vi "Quick Test.vi"() -> ()   [LabVIEW 2010]
uses:
  <vilib>/SwitchExecutive/nise.llb/niSE Multiconnect Mode Enum.ctl
panel:
  in  "Load All Channels":bool
  in  "DMM to DVDD":bool
  in  "SMU1 to VRECT":bool
  in  "stop":bool
  in  "SMU3 to VBAT + BATT SIM":bool
  in  "SMU3 to VBAT":bool
  in  "JTAG DVDD POWER":bool
  in  "JTAG DATA":bool
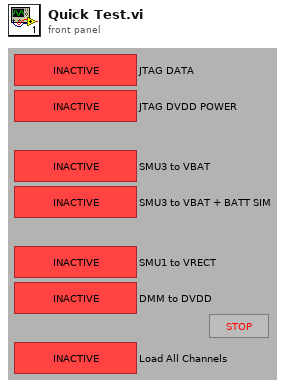
[diagram p1: front panel]
types:
  T1 = typedef "niSE Multiconnect Mode Enum.ctl" = i32
  T2 = typedef "niSE SessionRefnum.ctl" = refnum<k1>
  T3 = enum16{"--Disconnect All--", "Connect PulseGen to CH1", "Connect PulseGen to CH2", "Connect PulseGen to CH3", "Connect PulseGen to CH4", "Connect PulseGen to CH5", "Connect PulseGen to CH6", "Connect PulseGen to CH7", "Connect PulseGen to CH8", "Connect PulseGen to CH9", "Connect PulseGen to CH10", "Connect PulseGen to CH11", "Connect PulseGen to CH12", "Connect PulseGen to CH13", "Connect PulseGen to CH14", "Connect PulseGen to CH15", "Connect PulseGen to CH16", "Connect PulseGen to CH17", "Connect PulseGen to CH18", "Connect PulseGen to CH19", "Connect PulseGen to CH20", "Connect PulseGen to CH21", "Connect PulseGen to CH22", "Connect PulseGen to CH23", "Connect PulseGen to CH24", "Connect PulseGen to CH25", "Set MAG_SW", "Set Dynamic Load", "Set Expansion Trigger", "Trigger Positive Pulse", "Trigger Negative Pulse", "Set MSP Magic Pin", "Set BAT_EN", "Connect MSP_ACLK to CTR", "Connect MSP_MCLK to CTR", "Connect MSP_DIG_TST_OUT to CTR", "Connect STIM_SCK to CTR", "Connect STIM_CLK to CTR", "Connect SMU2 to Magnet", "Magnet Enable", "Cap Short", "Connect Positive Pulse to Pulse Bus", "Connect Negative Pulse to Pulse Bus", "Connect JTAG", "Connect JTAG DVDD Power", "RF Attach", "Connect SMU3 to VBAT", "Connect SMU3 Soft Start", "Connect ARB to Charge Coil", "Connect ARB to Matrix", "Connect CTR to Matrix", "DMM_I Short", "DMM_I 1000 Ohm", "DMM_I 100 Ohm", "DMM_I 10 Ohm", "Connect CH25 to DUT GND"}
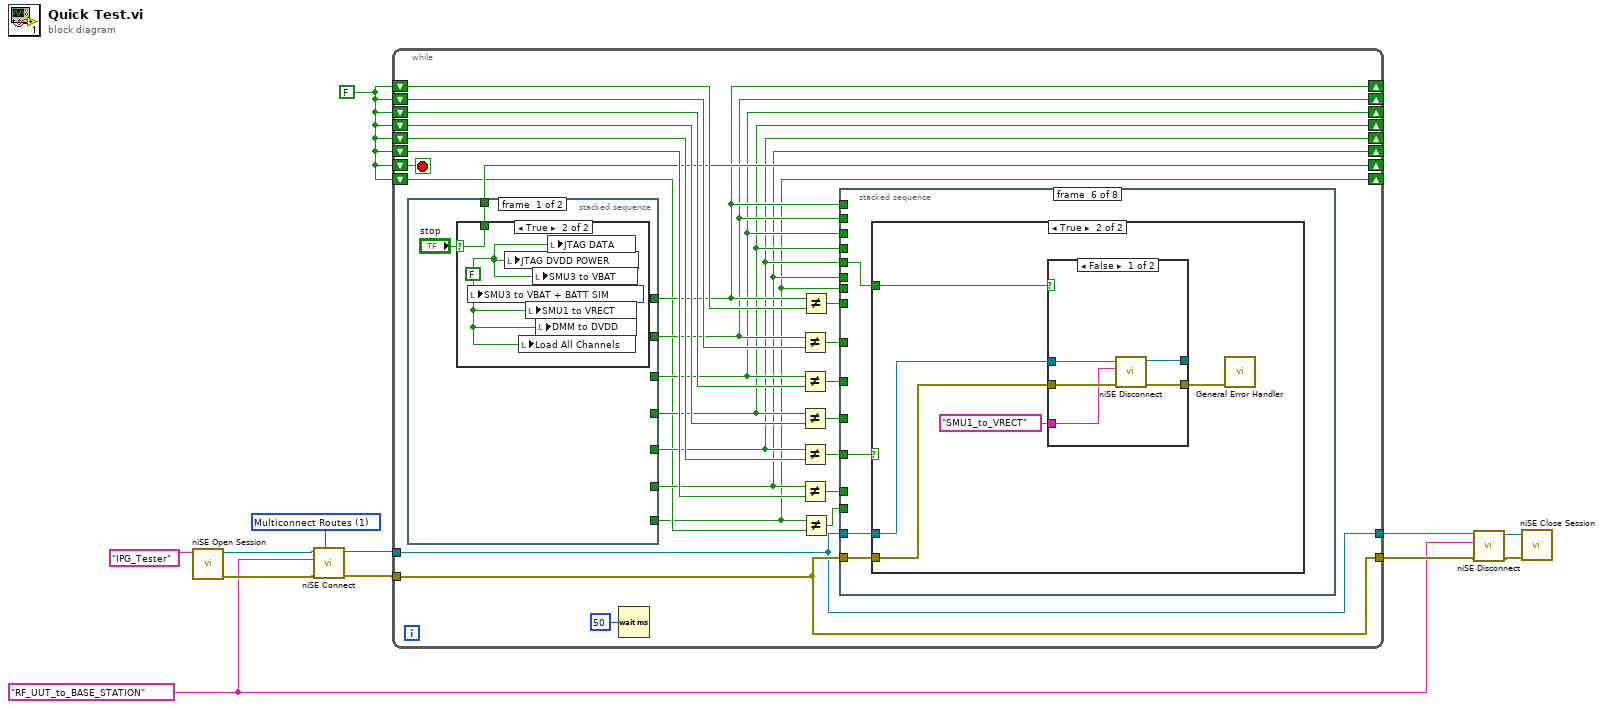
[diagram p0: block diagram]
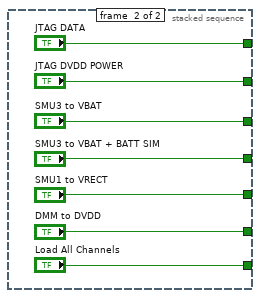
[diagram p3: hidden frame]
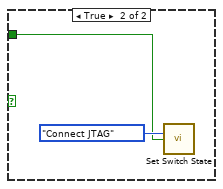
[diagram p6: hidden frame]
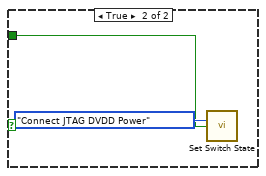
[diagram p8: hidden frame]
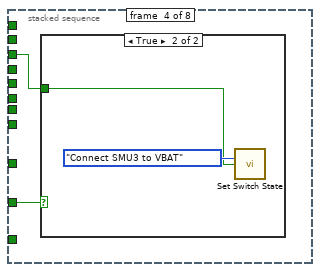
[diagram p9: hidden frame]
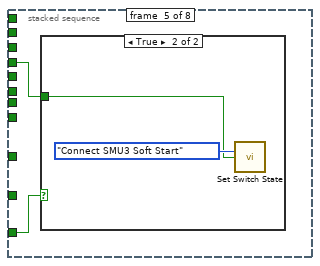
[diagram p11: hidden frame]
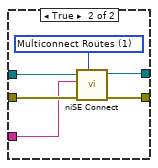
[diagram p14: hidden frame]
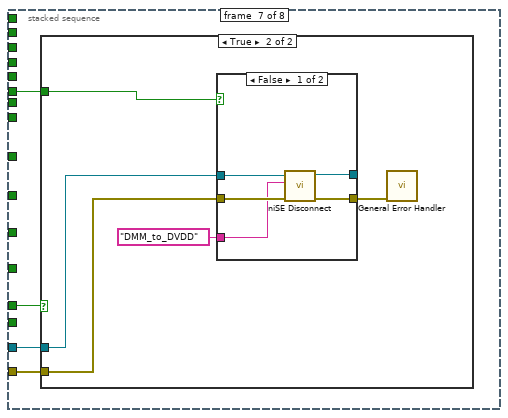
[diagram p15: hidden frame]
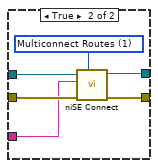
[diagram p17: hidden frame]
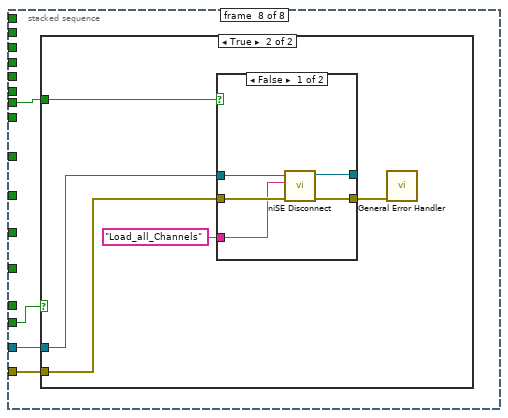
[diagram p18: hidden frame]
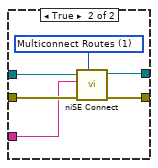
[diagram p20: hidden frame]
diagram:
  w1 = "RF_UUT_to_BASE_STATION" ("Connection Specification (\"\")")
  w10 = T1 1 items=["Use Default Mode"=-1, "Multiconnect Routes"=1, "No Multiconnect"=0] ("Multiconnect Mode (Use Default Mode)")
  w11 = FALSE
  n1 = call <vilib>:"niSE Open Session.vi"("Virtual Device Name (SwitchConfiguration1)"="IPG_Tester") -> ("error out"=w3:errorcluster, "NISE Session (out)"=w5:T2)  [unwired: 5 in]
  n2 = call <vilib>:"niSE Connect.vi"("Multiconnect Mode (Use Default Mode)"=w10, "error in (no error)"=w3, "Connection Specification (\"\")"=w1, "NISE Session (in)"=w5) -> ("error out"=w2:errorcluster, "NISE Session (out)"=w4:T2)  [unwired: 6 in]
  n3 = while {
    shift-right: [w21] -> _
    shift-left: w11 -> [w38]
    shift-right: [w20] -> _
    shift-left: w11 -> [w37]
    shift-right: [w19] -> _
    shift-left: w11 -> [w36]
    shift-right: [w18] -> _
    shift-left: w11 -> [w35]
    shift-right: [w17] -> _
    shift-left: w11 -> [w27]
    shift-right: [w16] -> _
    shift-left: w11 -> [w26]
    tunnel: w4 -> [w24]
    tunnel: w2 -> [w25]
    tunnel: [w24] -> w9
    tunnel: [w25] -> w7
    shift-right: [w22] -> _
    shift-left: w11 -> [w23]
    shift-right: [w13] -> _
    shift-left: w11 -> [w15]
    stop <- w23 stop-if-true
    n4 = stacked-sequence {
      tunnel: [w39 _] -> w22
      tunnel: [_ "JTAG DATA"] -> w21
      tunnel: [_ "JTAG DVDD POWER"] -> w20
      tunnel: [_ "SMU3 to VBAT"] -> w19
      tunnel: [_ "SMU3 to VBAT + BATT SIM"] -> w18
      tunnel: [_ "SMU1 to VRECT"] -> w17
      tunnel: [_ "DMM to DVDD"] -> w16
      tunnel: [_ "Load All Channels"] -> w13
      frame #0 {
        n5 = case shown="True" "stop" {
          selector: "stop" -> [w41 w43]
          tunnel: [w41 w43] -> w39
          frame False {
          }
          frame True {
            w42 = FALSE
            n6 = local write "SMU3 to VBAT + BATT SIM"(w42) -> ()
            n7 = local write "JTAG DVDD POWER"(w42) -> ()
            n8 = local write "Load All Channels"(w42) -> ()
            n9 = local write "SMU1 to VRECT"(w42) -> ()
            n10 = local write "SMU3 to VBAT"(w42) -> ()
            n11 = local write "DMM to DVDD"(w42) -> ()
            n12 = local write "JTAG DATA"(w42) -> ()
          }
        }
      }
      frame #1 {
      }
    }
    n13 = Wait (ms)(milliseconds to wait=u32 50) -> ()  [unwired: 1 out]
    n14 = Not Equal?(x=w20, y=w37) -> (x != y?=w33:bool)
    n15 = Not Equal?(x=w19, y=w36) -> (x != y?=w32:bool)
    n16 = Not Equal?(x=w18, y=w35) -> (x != y?=w31:bool)
    n17 = Not Equal?(x=w17, y=w27) -> (x != y?=w29:bool)
    n18 = Not Equal?(x=w16, y=w26) -> (x != y?=w28:bool)
    n19 = Not Equal?(x=w21, y=w38) -> (x != y?=w34:bool)
    n20 = Not Equal?(x=w13, y=w15) -> (x != y?=w14:bool)
    n21 = stacked-sequence {
      tunnel: w18 -> [_ _ _ _ w63 _ _ _]
      tunnel: w19 -> [_ _ _ w59 _ _ _ _]
      tunnel: w20 -> [_ _ w56 _ _ _ _ _]
      tunnel: w21 -> [_ w52 _ _ _ _ _ _]
      tunnel: w34 -> [_ w51 _ _ _ _ _ _]
      tunnel: w33 -> [_ _ w55 _ _ _ _ _]
      tunnel: w32 -> [_ _ _ w60 _ _ _ _]
      tunnel: w31 -> [_ _ _ _ w64 _ _ _]
      tunnel: w29 -> [_ _ _ _ _ w70 _ _]
      tunnel: w28 -> [_ _ _ _ _ _ w89 _]
      tunnel: w17 -> [_ _ _ _ _ w69 _ _]
      tunnel: w16 -> [_ _ _ _ _ _ w90 _]
      tunnel: w24 -> [_ _ _ _ _ w67 w88 w110]
      tunnel: w25 -> [_ _ _ _ _ w68 w87 w109]
      tunnel: w14 -> [_ _ _ _ _ _ _ w108]
      tunnel: w13 -> [_ _ _ _ _ _ _ w107]
      frame #0 {
      }
      frame #1 {
        n22 = case shown="False" w51 {
          tunnel: w52 -> [_ w53]
          frame False {
          }
          frame True {
            n23 = call "Set Switch State.vi"("Action"=T3."Connect JTAG", "State"=w53) -> ()  [unwired: 13 in, 1 out]
          }
        }
      }
      frame #2 {
        n24 = case shown="False" w55 {
          tunnel: w56 -> [_ w57]
          frame False {
          }
          frame True {
            n25 = call "Set Switch State.vi"("Action"=T3."Connect JTAG DVDD Power", "State"=w57) -> ()  [unwired: 13 in, 1 out]
          }
        }
      }
      frame #3 {
        n26 = case shown="True" w60 {
          tunnel: w59 -> [_ w61]
          frame False {
          }
          frame True {
            n27 = call "Set Switch State.vi"("Action"=T3."Connect SMU3 to VBAT", "State"=w61) -> ()  [unwired: 13 in, 1 out]
          }
        }
      }
      frame #4 {
        n28 = case shown="True" w64 {
          tunnel: w63 -> [_ w65]
          frame False {
          }
          frame True {
            n29 = call "Set Switch State.vi"("Action"=T3."Connect SMU3 Soft Start", "State"=w65) -> ()  [unwired: 13 in, 1 out]
          }
        }
      }
      frame #5 {
        n30 = case shown="True" w70 {
          tunnel: w69 -> [_ w75]
          tunnel: w68 -> [_ w73]
          tunnel: w67 -> [_ w72]
          frame False {
          }
          frame True {
            n31 = case shown="False" w75 {
              tunnel: w72 -> [w80 w84]
              tunnel: [w79 w86] -> w71
              tunnel: w73 -> [w78 w85]
              tunnel: [w77 w83] -> _
              tunnel: "SMU1_to_VRECT" ("Virtual Device Name (SwitchConfiguration1)") -> [w76 w82]
              frame False {
                n32 = call <vilib>:"niSE Disconnect.vi"("error in (no error)"=w78, "Disconnection Specification (\"\")"=w76, "NISE Session (in)"=w80) -> ("error out"=w79:errorcluster, "NISE Session (out)"=w77:T2)  [unwired: 3 in]
              }
              frame True {
                w81 = T1 1 items=["Use Default Mode"=-1, "Multiconnect Routes"=1, "No Multiconnect"=0] ("Multiconnect Mode (Use Default Mode)")
                n33 = call <vilib>:"niSE Connect.vi"("Multiconnect Mode (Use Default Mode)"=w81, "error in (no error)"=w85, "Connection Specification (\"\")"=w82, "NISE Session (in)"=w84) -> ("error out"=w86:errorcluster, "NISE Session (out)"=w83:T2)  [unwired: 6 in]
              }
            }
            n34 = call <vilib>:"General Error Handler.vi"("error in (no error)"=w71) -> ()  [unwired: 10 in, 5 out]
          }
        }
      }
      frame #6 {
        n35 = case shown="True" w89 {
          tunnel: w90 -> [_ w95]
          tunnel: w88 -> [_ w93]
          tunnel: w87 -> [_ w92]
          frame False {
          }
          frame True {
            n36 = case shown="False" w95 {
              tunnel: w93 -> [w100 w104]
              tunnel: [w99 w106] -> w91
              tunnel: w92 -> [w98 w105]
              tunnel: [w97 w103] -> _
              tunnel: "DMM_to_DVDD" ("Virtual Device Name (SwitchConfiguration1)") -> [w96 w102]
              frame False {
                n37 = call <vilib>:"niSE Disconnect.vi"("error in (no error)"=w98, "Disconnection Specification (\"\")"=w96, "NISE Session (in)"=w100) -> ("error out"=w99:errorcluster, "NISE Session (out)"=w97:T2)  [unwired: 3 in]
              }
              frame True {
                w101 = T1 1 items=["Use Default Mode"=-1, "Multiconnect Routes"=1, "No Multiconnect"=0] ("Multiconnect Mode (Use Default Mode)")
                n38 = call <vilib>:"niSE Connect.vi"("Multiconnect Mode (Use Default Mode)"=w101, "error in (no error)"=w105, "Connection Specification (\"\")"=w102, "NISE Session (in)"=w104) -> ("error out"=w106:errorcluster, "NISE Session (out)"=w103:T2)  [unwired: 6 in]
              }
            }
            n39 = call <vilib>:"General Error Handler.vi"("error in (no error)"=w91) -> ()  [unwired: 10 in, 5 out]
          }
        }
      }
      frame #7 {
        n40 = case shown="True" w108 {
          tunnel: w107 -> [_ w115]
          tunnel: w110 -> [_ w113]
          tunnel: w109 -> [_ w112]
          frame False {
          }
          frame True {
            n41 = case shown="False" w115 {
              tunnel: w113 -> [w120 w124]
              tunnel: [w119 w126] -> w111
              tunnel: w112 -> [w118 w125]
              tunnel: [w117 w123] -> _
              tunnel: "Load_all_Channels" ("Virtual Device Name (SwitchConfiguration1)") -> [w116 w122]
              frame False {
                n42 = call <vilib>:"niSE Disconnect.vi"("error in (no error)"=w118, "Disconnection Specification (\"\")"=w116, "NISE Session (in)"=w120) -> ("error out"=w119:errorcluster, "NISE Session (out)"=w117:T2)  [unwired: 3 in]
              }
              frame True {
                w121 = T1 1 items=["Use Default Mode"=-1, "Multiconnect Routes"=1, "No Multiconnect"=0] ("Multiconnect Mode (Use Default Mode)")
                n43 = call <vilib>:"niSE Connect.vi"("Multiconnect Mode (Use Default Mode)"=w121, "error in (no error)"=w125, "Connection Specification (\"\")"=w122, "NISE Session (in)"=w124) -> ("error out"=w126:errorcluster, "NISE Session (out)"=w123:T2)  [unwired: 6 in]
              }
            }
            n44 = call <vilib>:"General Error Handler.vi"("error in (no error)"=w111) -> ()  [unwired: 10 in, 5 out]
          }
        }
      }
    }
  }
  n45 = call <vilib>:"niSE Disconnect.vi"("error in (no error)"=w7, "Disconnection Specification (\"\")"=w1, "NISE Session (in)"=w9) -> ("error out"=w6:errorcluster, "NISE Session (out)"=w8:T2)  [unwired: 3 in]
  n46 = call <vilib>:"niSE Close Session.vi"("error in (no error)"=w6, "NISE Session (in)"=w8) -> ()  [unwired: 5 in, 1 out]
